vi "InitPreprocSession.vi"(8 "error in (no error)":errorcluster, 11 "Python.lvclass":refnum<class "Python.lvclass">) -> (0 "error out":errorcluster, 3 "Python.lvclass":refnum<class "Python.lvclass">)   [LabVIEW 2020, in "Python.lvclass"]
uses:
  Python.lvclass
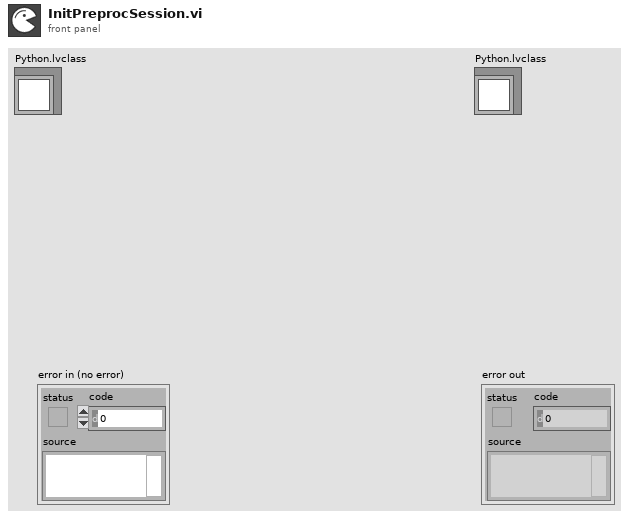
[diagram p1: front panel]
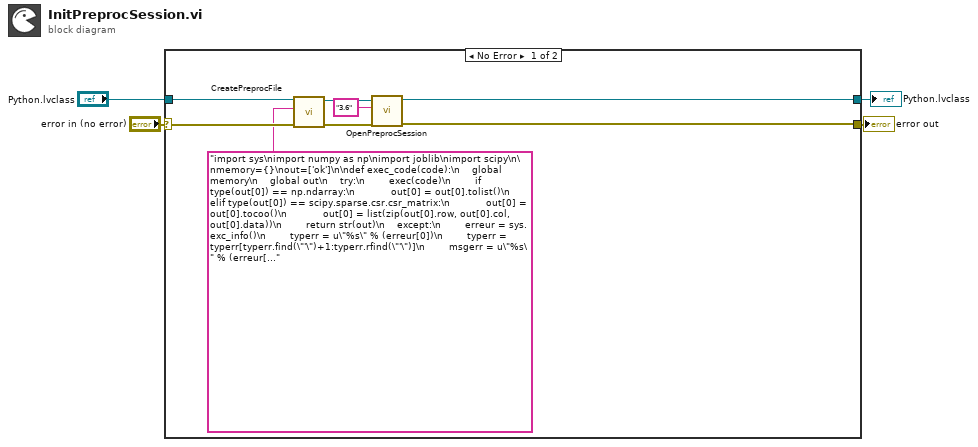
[diagram p0: block diagram]
diagram:
  n1 = case shown="No Error" "error in (no error)" {
    selector: "error in (no error)" -> [w9 w14]
    tunnel: [w6 w14] -> w3
    tunnel: [w7 w13] -> w1
    tunnel: "Python.lvclass" -> [w12 w13]
    frame No Error {
      n2 = call-dynamic "CreatePreprocFile.vi"("error in (no error)"=w9, "Python Instruction"="import sys\nimport numpy as np\nimport joblib\nimport scipy\n\nmemory={}\nout=['ok']\n\ndef exec_code(code):\n    global memory\n    global out\n    try:\n        exec(code)\n        if type(out[0]) == np.ndarray:\n            out[0] = out[0].tolist()\n        elif type(out[0]) == scipy.sparse.csr.csr_matrix:\n            out[0] = out[0].tocoo()\n            out[0] = list(zip(out[0].row, out[0].col, out[0].data))\n        return str(out)\n    except:\n        erreur = sys.exc_info()\n        typerr = u\"%s\" % (erreur[0])\n        typerr = typerr[typerr.find(\"'\")+1:typerr.rfind(\"'\")]\n        msgerr = u\"%s\" % (erreur[1])\n        message = str('/!\\\\ {0} : {1}'. format(typerr,msgerr))\n        return message \n    \n\ndef save_model(UserModelName=str,path=str,Save_name=str):\n    try:\n        filename=path+'\\{}.gz'.format(Save_name)\n        joblib.dump(memory[UserModelName],filename=filename)\n        return filename\n    except:\n        erreur = sys.exc_info()\n        typerr = u\"%s\" % (erreur[0])\n        typerr = typerr[typerr.find(\"'\")+1:typerr.rfind(\"'\")]\n        msgerr = u\"%s\" % (erreur[1])\n        message = str('/!\\\\ {0} : {1}'. format(typerr,msgerr))\n        return message \n    \n\ndef load_model(UserModelName=str,file=str):\n\n    try:\n        memory[UserModelName]=joblib.load(filename=file) \n        return str(memory[UserModelName])\n    except:\n        erreur = sys.exc_info()\n        typerr = u\"%s\" % (erreur[0])\n        typerr = typerr[typerr.find(\"'\")+1:typerr.rfind(\"'\")]\n        msgerr = u\"%s\" % (erreur[1])\n        message = str('/!\\\\ {0} : {1}'. format(typerr,msgerr))\n        return message \n    \n\n\ndef get_attribute(UserModelName=str):\n\n    try:\n        attrib=[]\n        value =[]\n        Dir=memory[UserModelName].__dir__()\n\n        for i in Dir:\n            if (i[0]!='_' and i[-1]=='_'):\n                attrib.append(i)\n                try : \n                    if type(eval(\"memory['\"+UserModelName+\"'].\"+i)) == np.ndarray:\n                        value.append(str(eval(\"memory['\"+UserModelName+\"'].\"+i).tolist()))\n                    elif type(eval(\"memory['\"+UserModelName+\"'].\"+i)) == dict:\n                        value.append(str(eval(\"memory['\"+UserModelName+\"'].\"+i))[1:-1])\n                    else:\n                        value.append(str(eval(\"memory['\"+UserModelName+\"'].\"+i)))\n                except AttributeError:\n                    erreur = sys.exc_info()\n                    typerr = u\"%s\" % (erreur[0])\n                    typerr = typerr[typerr.find(\"'\")+1:typerr.rfind(\"'\")]\n                    msgerr = u\"%s\" % (erreur[1])\n                    message = '/!\\ {0} : {1}'. format(typerr,msgerr)\n                    value.append(message)\n                    \n        s={}\n        s=dict(zip(attrib,value))\n        return str(s)\n    except:\n        erreur = sys.exc_info()\n        typerr = u\"%s\" % (erreur[0])\n        typerr = typerr[typerr.find(\"'\")+1:typerr.rfind(\"'\")]\n        msgerr = u\"%s\" % (erreur[1])\n        message = str('/!\\\\ {0} : {1}'. format(typerr,msgerr))\n        return message\n\n    \ndef get_help(UserModelName=str):\n    try:\n        return str(memory[UserModelName].__doc__)\n    except:\n        erreur = sys.exc_info()\n        typerr = u\"%s\" % (erreur[0])\n        typerr = typerr[typerr.find(\"'\")+1:typerr.rfind(\"'\")]\n        msgerr = u\"%s\" % (erreur[1])\n        message = str('/!\\\\ {0} : {1}'. format(typerr,msgerr))\n        return message \n    ", "Python in"=w12) -> ("error out"=w8:errorcluster, "Python out"=w11:refnum<class "Python.lvclass">)  [unwired: 7 in]
      n3 = call-dynamic "OpenPreprocSession.vi"("error in (no error)"=w8, "Python version"="3.6", "Python in"=w11) -> ("error out"=w6:errorcluster, "Python out"=w7:refnum<class "Python.lvclass">)  [unwired: 7 in]
    }
    frame Error {
    }
  }
  "error out" <- w3
  "Python.lvclass" <- w1
